vi "Actor Core.vi"(8 "error in":errorcluster, 11 "ViewableChart In":refnum<class "ViewManagerDefaultLayout.lvclass">) -> (0 "error out":errorcluster, 3 "Actor out":refnum<class "Actor.lvclass">)   [LabVIEW 2017, in "ViewManagerDefaultLayout.lvclass"]
doc: "(<B>Filename</B>: Actor Framework.lvlib:Actor.lvclass:Actor Core.vi)\n\nReceives messages to the actor, reacts to them, and initiates any error handling that may shut the actor down.\n\nDescendant classes may override this VI to append parallel tasks for the actor to complete while it handles messages. Overrides use the Call Parent Method node.\n\n<License>\nCopyright © 2017 Composed Systems, LLC | All rights reserved\nwww.composed.io\n\nAuthor: Ethan Stern <ethan.stern@composed.io>\n\nThis software is provided \"AS IS\" WITHOUT WARRANTIES, either express or implied, AND IS FOR EDUCATIONAL PURPOSES ONLY.\n</License>MVA Framework 1.7.0.33\nEthan Stern - Composed Systems\nCopyright (c) 2018, Composed Systems"
uses:
  <vilib>/gpm_packages/@cs/example/Dynamic Viewables/ViewManagerDefaultLayout/ViewManagerDefaultLayout.lvclass
  <vilib>/ActorFramework/Actor/Actor.lvclass
  <vilib>/gpm_packages/@cs/example/Dynamic Viewables/ViewManagerDefaultLayout/ViewManagerDefaultLayout.lvclass/ViewManagerDefaultLayout.ctl
  <vilib>/gpm_packages/@cs/mva-viewable/Source/IViewManager/IViewManager/IViewManager.lvclass
  <vilib>/gpm_packages/@cs/mva-viewable/Source/IViewable/ProtectedSubpanel/ProtectedSubpanel.lvclass
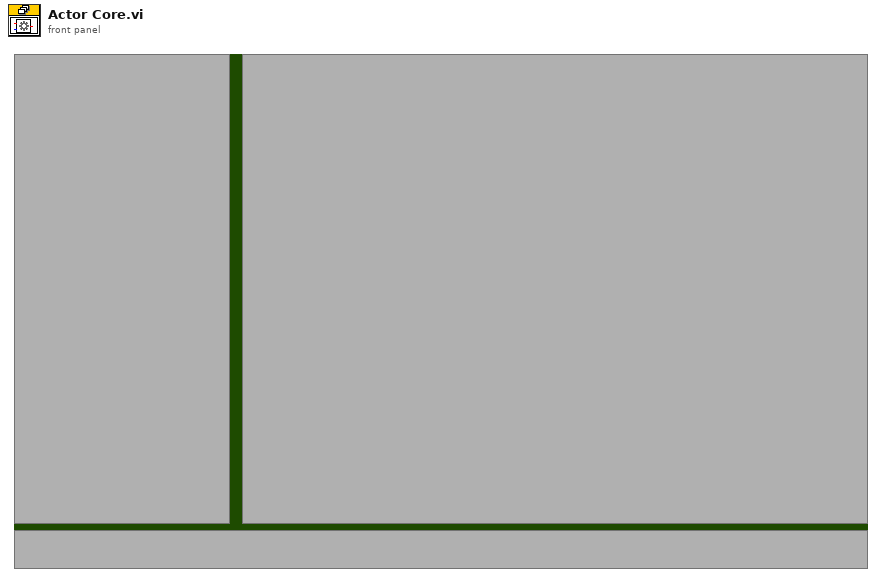
[diagram p1: front panel]
types:
  T1 = typedef "IViewable.lvlib/ProtectedSubpanel.lvclass/Protected Subpanel Reference.ctl" = refnum<data-value>
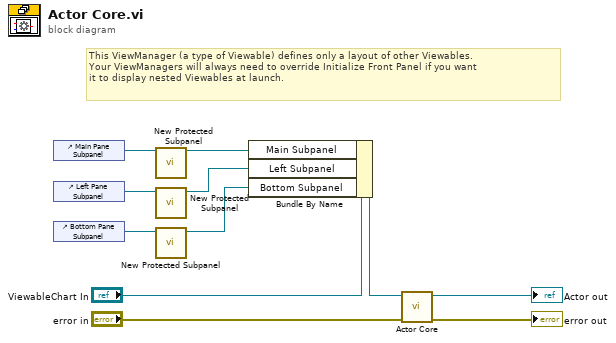
[diagram p0: block diagram]
diagram:
  # "This ViewManager (a type of Viewable) defines only a layout of other Viewables.\nYour ViewManagers will always need to override Initialize Front Panel if you want\nit to display nested Viewables at launch."
  n1 = control-ref of="Main Pane Subpanel"() -> (w6:refnum<vi>)
  n2 = control-ref of="Left Pane Subpanel"() -> (w4:refnum<vi>)
  n3 = control-ref of="Bottom Pane Subpanel"() -> (w3:refnum<vi>)
  n4 = call <vilib>:"New Protected Subpanel.vi"("SubPnl Refnum"=w6) -> ("Protected Subpanel"=w5:T1)  [unwired: 9 in, 1 out]
  n5 = call <vilib>:"New Protected Subpanel.vi"("SubPnl Refnum"=w4) -> ("Protected Subpanel"=w2:T1)  [unwired: 9 in, 1 out]
  n6 = call <vilib>:"New Protected Subpanel.vi"("SubPnl Refnum"=w3) -> ("Protected Subpanel"=w1:T1)  [unwired: 9 in, 1 out]
  n7 = Bundle By Name(cluster="ViewableChart In", "Main Subpanel"=w5, "Left Subpanel"=w2, "Bottom Subpanel"=w1) -> (w7:refnum<class "ViewManagerDefaultLayout.lvclass">)
  n8 = call-parent "Actor Core.vi"("error in"="error in", "IViewable In"=w7) -> ("error out"=→"error out":errorcluster, "Actor out"=→"Actor out":refnum<class "Actor.lvclass">)  [unwired: 8 in]
